vi "Calibrate Channel.vi"(4 "Ctrl Name":string, 6 "Row":i32, 8 "error in (no error)":errorcluster, 9 "Hdr Names":T3[](array[typedef]), 10 "Chassis Name":string, 11 "Voltage in":refnum<class "Voltage.lvclass">) -> (0 "error out":errorcluster, 2 "Cell Contents":T1[](array[typedef]))   [LabVIEW 2012, in "Measurement Channels.lvlib" / "Voltage.lvclass"]
uses:
  Voltage.lvclass
  Common/Controls/HeaderNames.ctl
  SubVIs Table/Custom Ctls Table/ge_CellContents.ctl
  <vilib>/Utility/miscctls.llb/LVPoint32TypeDef.ctl
  <vilib>/DAQmx/read.llb/DAQmx Read (Analog 1D DBL 1Chan NSamp).vi
  Class Channel/Read Device.vi
  <vilib>/DAQmx/configure/timing.llb/DAQmx Timing (Sample Clock).vi
  <vilib>/Analysis/baseanly.llb/Mean (DBL).vi
  <vilib>/DAQmx/miscellaneous.llb/DAQmx Fill In Error Info.vi
  <resource>/objmgr/daqmx.rc
  <vilib>/Analysis/NI_AALBase.lvlib
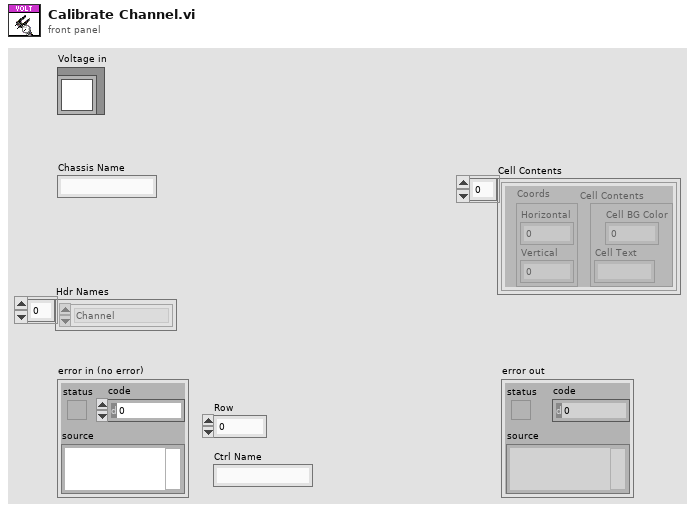
[diagram p1: front panel]
types:
  T1 = typedef "ge_CellContents.ctl" = cluster{"Cell Contents":cluster{"Cell Text":string, "Cell BG Color":u32}, "Coords":T2}
  T2 = typedef "LVPoint32TypeDef.ctl" = cluster{"Horizontal":i32, "Vertical":i32}
  T3 = typedef "HeaderNames.ctl" = enum16{"Channel", "Device", "Spacer", "Description", "MB", "Range", "Terminal", "Coupling", "Thresh (V)", "Pulse/Rev", "Slope", "Min EU", "Min RPM", "mV/EU", "Iex", "Temp Units", "Type", "CJC Src", "CJC Val", "Ro", "Wire Cfg", "Strain Mode", "Vex", "Bridge Type", "GF", "Gauge Res", "Poisson", "Lead Res", "Init Strain", "GAF", "Scale", "Offset", "Unit (EU)", "dB?", "dB Ref", "Cal Mag", "Cal Units", "Max Temp", "Min Temp", "Max Strain", "Min Strain"}
  T4 = cluster{cluster{"Float String":string, "Coerced":u32}, cluster{"Row":i32, "index of element":i32}}
  T5 = cluster{cluster{"Float String":string, "Coerced":u32}, cluster{"Row":i32, "index of element":i32}}[]
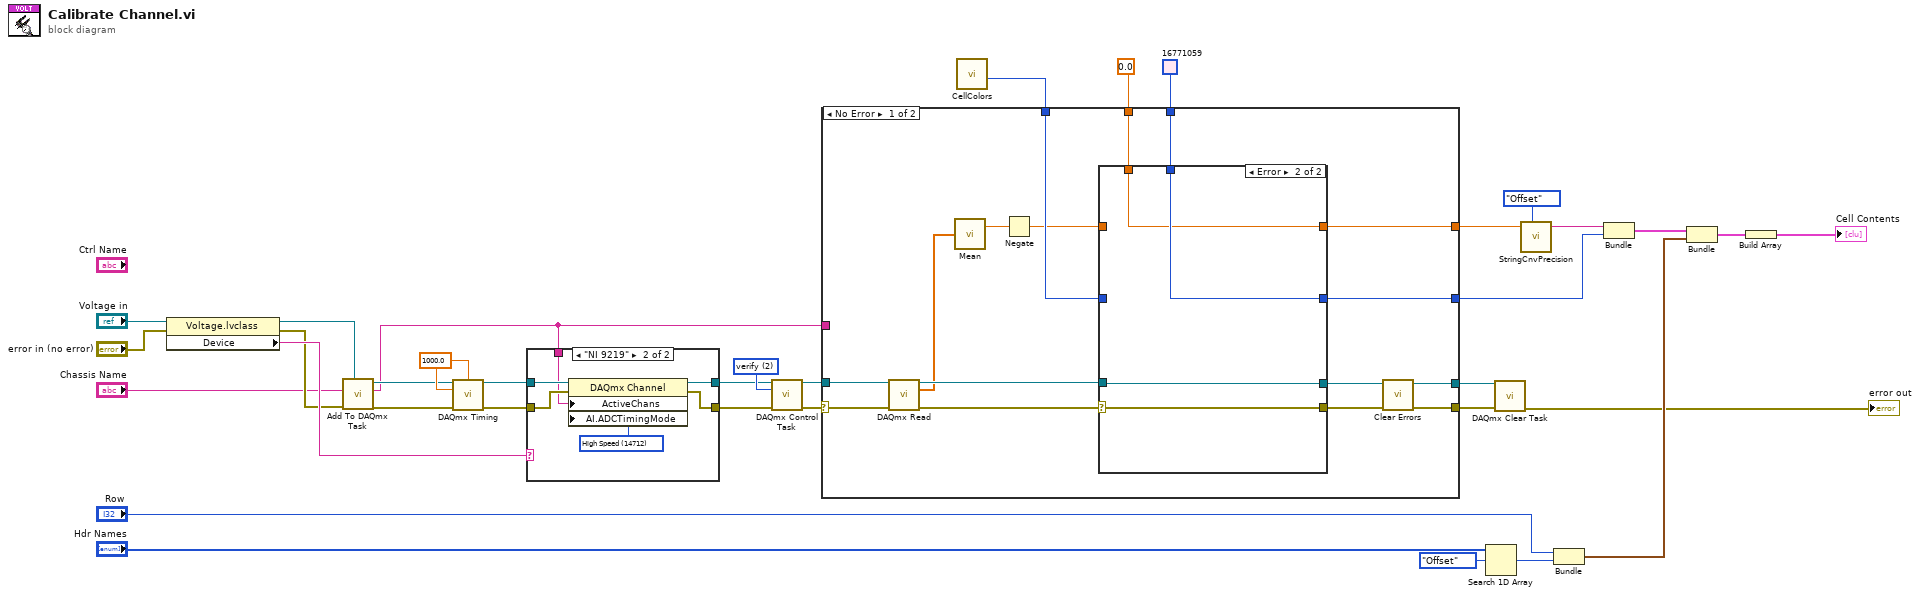
[diagram p0: block diagram]
diagram:
  w32 = 2 items=["verify"=2, "reserve"=4, "commit"=3, "unreserve"=5, "abort"=6] ("action")
  w27 = 1000.0 ("rate")
  n1 = property class="Voltage.lvclass"(reference="Voltage in", error in="error in (no error)") -> (reference out=w12:refnum<class "Voltage.lvclass">, error out=w8:errorcluster, "Device"=w9:string)
  n2 = call-dynamic "Add To DAQmx Task.vi"("Voltage in"=w12, "error in (no error)"=w8, "Chassis Name"="Chassis Name") -> ("error out"=w10:errorcluster, "Phys Chan Added"=w7:string, "task out"=w11:refnum<k21>)  [unwired: 6 in]
  n3 = call-poly <vilib>:"DAQmx Timing.vi"("task/channels in"=w11, "samples per channel"=w27, "rate"=w27, "error in"=w10) -> ("task out"=w26:refnum<k21>, "error out"=w23:errorcluster)  [unwired: 10 in]
  n4 = case shown="\"NI 9219\"" w9 {
    tunnel: w26 -> [w37 w42]
    tunnel: [w37 w41] -> w25
    tunnel: [w36 w40] -> w24
    tunnel: w23 -> [w36 w39]
    tunnel: w7 -> [_ w38]
    frame Default {
    }
    frame "NI 9219" {
      w43 = 14712 items=["High Resolution"=10195, "High Speed"=14712, "Best 50 Hz Rejection"=14713, "Best 60 Hz Rejection"=14714, "Custom"=10137] ("AI.ADCTimingMode")
      n5 = property class="DAQmx Channel"(reference=w42, error in=w39, "ActiveChans"=w38, "AI.ADCTimingMode"=w43) -> (reference out=w41:refnum<k21>, error out=w40:errorcluster)
    }
  }
  n6 = call <vilib>:"DAQmx Control Task.vi"("task/channels in"=w25, "action"=w32, "error in"=w24) -> ("task out"=w33:refnum<k21>, "error out"=w31:errorcluster)  [unwired: 11 in]
  n7 = call "CellColors.vi"() -> ("Coerced"=w28:u32)  [unwired: 8 in, 3 out]
  n8 = case shown="No Error" w31 {
    selector: w31 -> [w50 w70]
    tunnel: [w58 w69] -> w35
    tunnel: [w53 w70] -> w34
    tunnel: w33 -> [w51 w69]
    tunnel: [w57 w68] -> w15
    tunnel: sgl 0.0 -> [w56 w68]
    tunnel: [w55 w67] -> w14
    tunnel: u32 16771059 -> [w54 w67]
    tunnel: w28 -> [w46 _]
    tunnel: w7 -> [_ _]
    frame No Error {
      n9 = call-poly <vilib>:"DAQmx Read.vi"("task/channels in"=w51, "error in"=w50) -> ("task out"=w49:refnum<k21>, "data"=w47:dbl[], "error out"=w48:errorcluster)  [unwired: 11 in]
      n10 = call-poly <vilib>:"Mean.vi"("X"=w47) -> ("mean"=w45:dbl)  [unwired: 1 out]
      n11 = Negate(x=w45) -> (-x=w44:dbl)
      n12 = case shown="Error" w48 {
        selector: w48 -> [w62 w64]
        tunnel: [w62 w64] -> w52
        tunnel: w49 -> [w61 w65]
        tunnel: [w61 w65] -> w58
        tunnel: w46 -> [w60 _]
        tunnel: [w60 w66] -> w55
        tunnel: w54 -> [_ w66]
        tunnel: [w59 w63] -> w57
        tunnel: w56 -> [_ w63]
        tunnel: w44 -> [w59 _]
        frame No Error {
        }
        frame Error {
        }
      }
      n13 = call <vilib>:"Clear Errors.vi"("error in (no error)"=w52) -> ("error out"=w53:errorcluster)  [unwired: 6 in]
    }
    frame Error {
    }
  }
  n14 = Search 1D Array(1D array="Hdr Names", element=HeaderNames."Offset") -> (index of element=w21:i32)  [unwired: 1 in]
  n15 = call <vilib>:"DAQmx Clear Task.vi"("task in"=w35, "error in"=w34) -> ("error out"=→"error out":errorcluster)  [unwired: 13 in]
  n16 = call "StringCnvPrecision.vi"("Number"=w15, "Header"=HeaderNames."Offset") -> ("Float String"=w19:string)  [unwired: 5 in]
  n17 = Bundle("Row"="Row", "index of element"=w21) -> (w20:cluster{"Row":i32, "index of element":i32})  [unwired: 1 in]
  n18 = Bundle("Float String"=w19, "Coerced"=w14) -> (w22:cluster{"Float String":string, "Coerced":u32})  [unwired: 1 in]
  n19 = Bundle(w22, w20) -> (w18:T4)  [unwired: 1 in]
  n20 = Build Array(w18) -> (→"Cell Contents":T5)
